vi "Power Clear Request.vi"(8 "error in (no error)":errorcluster, 10 "Power Request Type":T1, 11 "Handle in":i64) -> (0 "error out":errorcluster, 2 "Success?":bool, 3 "Handle out":i64)   [LabVIEW 2016, in "Power Requests.lvlib"]
uses:
  <userlib>/Power-Requests-master/Power Requests.lvlib
  <userlib>/Power-Requests-master/Power Availabilty Requests/Type Defs/Power Request Type.ctl
  kernel32.dll
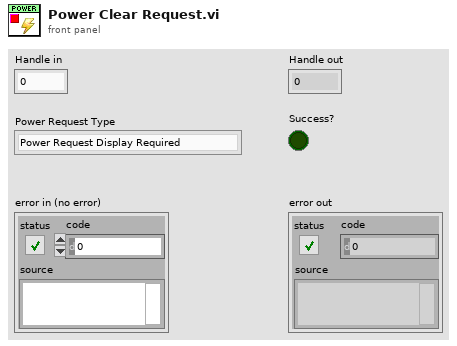
[diagram p1: front panel]
types:
  T1 = typedef "Power Requests.lvlib/Power Request Type.ctl" = enum32{"Power Request Display Required", "Power Request System Required", "Power Request Away Mode Required", "Power Request Execution Required"}
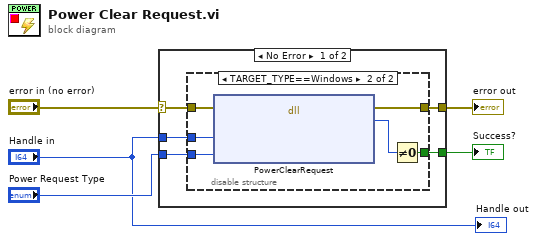
[diagram p0: block diagram]
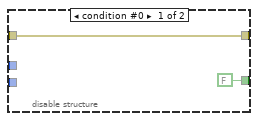
[diagram p2: hidden frame]
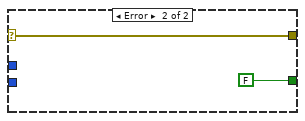
[diagram p3: hidden frame]
diagram:
  n1 = case shown="No Error" "error in (no error)" {
    selector: "error in (no error)" -> [w9 w20]
    tunnel: [w10 w20] -> w5
    tunnel: "Handle in" -> [w8 _]
    tunnel: "Power Request Type" -> [w7 _]
    tunnel: [w6 FALSE] -> w1
    frame No Error {
      n2 = disable-structure shown="TARGET_TYPE==Windows" {
        disable-tunnel: [w12 w18] -> w10
        disable-tunnel: w9 -> [w12 w17]
        disable-tunnel: w8 -> [_ w16]
        disable-tunnel: w7 -> [_ w15]
        disable-tunnel: [FALSE w13] -> w6
        frame condition #0 {
        }
        frame condition #1 (active) {
          n3 = dll-call lib="kernel32.dll" fn="PowerClearRequest"(error in=w17, "_In_ HANDLE"=w16, "_In_ POWER_REQUEST_TYPE"=w15) -> (error out=w18:errorcluster, "BOOL"=w14:i32)  [unwired: 4 in, 1 out]
          n4 = Not Equal To 0?(x=w14) -> (x != 0?=w13:bool)
        }
      }
    }
    frame Error {
    }
  }
  "error out" <- w5
  "Success?" <- w1
  "Handle out" <- "Handle in"
